vi "Test GIT Paths.vi"() -> ()   [LabVIEW 2020, in "UT_CICD.lvlib"]
uses:
  UT_CICD.lvlib
  Source/CICD.lvlib
panel:
  out "appended path":path
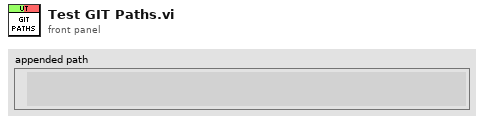
[diagram p1: front panel]
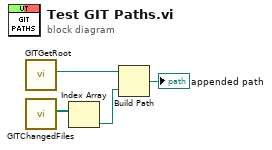
[diagram p0: block diagram]
diagram:
  n1 = call "GITGetRoot.vi"() -> ("path"=w3:path)  [unwired: 10 in, 1 out]
  n2 = call "GITChangedFiles.vi"() -> ("Files Changed"=w4:path[])  [unwired: 10 in, 1 out]
  n3 = Index Array(array=w4) -> (element=w2:path)  [unwired: 1 in]
  n4 = Build Path(base path=w3, name or relative path=w2) -> (appended path=→"appended path":path)
